vi "Intake.vi"   [LabVIEW 2014]
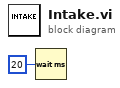
[diagram p0: block diagram]
diagram:
  n1 = Wait (ms)(milliseconds to wait=u32 20) -> ()  [unwired: 1 out]
